vi "Rayleigh Moments.vi"(10 "b":dbl=1.0) -> (0 "error":i32, 2 "variance":dbl=1.0, 3 "mean":dbl)   [LabVIEW 2017, in "NI_Gmath.lvlib"]
doc: "Returns the expected mean and variance of the random variate X, where X describes the selected distribution type. You must manually select the polymorphic instance to use."
uses:
  NI_Gmath.lvlib
  st_error_code.ctl
panel:
  # "Rayleigh Moments"
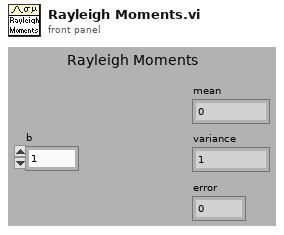
[diagram p1: front panel]
types:
  T1 = typedef "NI_Gmath.lvlib/st_error_code.ctl" = i32
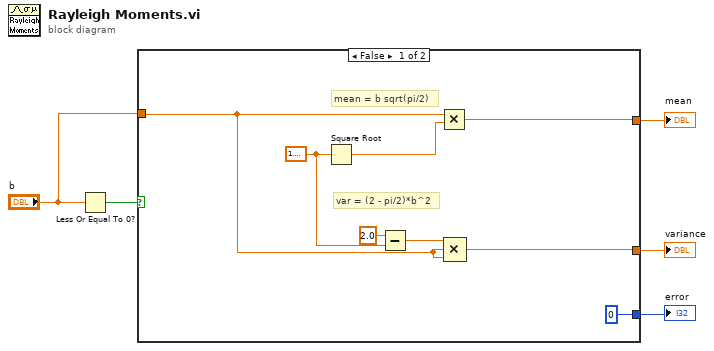
[diagram p0: block diagram]
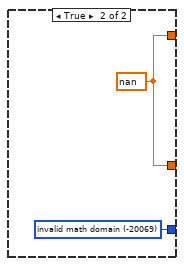
[diagram p2: hidden frame]
diagram:
  n1 = Less Or Equal To 0?(x="b") -> (x <= 0?=w3:bool)
  n2 = case shown="False" w3 {
    tunnel: "b" -> [w7 _]
    tunnel: [0 ("invalid math domain") w14] -> w5
    tunnel: [w11 w15] -> w4
    tunnel: [w6 w15] -> w1
    frame False {
      w9 = 1.5707963267948966
      # "var = (2 - pi/2)*b^2"
      # "mean = b sqrt(pi/2)"
      n3 = Square Root(x=w9) -> (sqrt(x)=w12:dbl)
      n4 = Subtract(x=2.0, y=w9) -> (x-y=w8:dbl)
      n5 = Multiply(x=w7, y=w12) -> (x*y=w11:dbl)
      n6 = Compound Arithmetic op=MULTIPLY(w8, w7, w7) -> (w6:dbl)
    }
    frame True {
      w14 = T1 -20069 items=["invalid math domain"=-20069, "Fourier interpolation size m >= n"=-20070, "empty array"=-20003] ("stat interp error code")
      w15 = nan
    }
  }
  "mean" <- w4
  "error" <- w5
  "variance" <- w1
